vi "Handle Incoming Packets.vi"(8 "error in (no error)":errorcluster, 9 "SessionMailbox":refnum<queue>, 10 "Incoming Packet":refnum<class "ControlPacket.lvclass">, 11 "Client in":refnum<class "Client.lvclass">) -> (0 "error out":errorcluster, 1 "SessionMailbox out":refnum<queue>, 2 "Outgoing":T1, 3 "Client out":refnum<class "Client.lvclass">)   [LabVIEW 2013, in "MQTT Client.lvlib" / "Client.lvclass"]
uses:
  Client.lvclass
  <vilib>/LabVIEW Open Source Project/MQTT Control Packets/Control Packets/ControlPacket/ControlPacket.lvclass
  MQTT_Base/Base Class/Response -- cluster.ctl
  Client.lvclass/Client.ctl
  <vilib>/LabVIEW Open Source Project/MQTT Control Packets/Control Packets/CONNACK/CONNACK.lvclass
  <vilib>/LabVIEW Open Source Project/MQTT Control Packets/Control Packets/CONNACK/Connect Return Code -- enum.ctl
  MQTT_Base/Base Class/MQTT_Base.lvclass
  <vilib>/LabVIEW Open Source Project/MQTT Control Packets/Control Packets/PUBREC/PUBREC.lvclass
  <vilib>/LabVIEW Open Source Project/MQTT Control Packets/Control Packets/PUBLISH/PUBLISH.lvclass
  <vilib>/LabVIEW Open Source Project/MQTT Control Packets/Control Packets/PUBCOMP/PUBCOMP.lvclass
  <vilib>/LabVIEW Open Source Project/MQTT Control Packets/Control Packets/ControlPacket/ControlPacket.lvclass/ControlPacket.ctl
  <vilib>/LabVIEW Open Source Project/MQTT Control Packets/Control Packets/SUBACK/SUBACK.lvclass
  <vilib>/LabVIEW Open Source Project/MQTT Control Packets/Control Packets/UNSUBACK/UNSUBACK.lvclass
  <vilib>/LabVIEW Open Source Project/MQTT Control Packets/Control Packets/PINGRESP/PINGRESP.lvclass
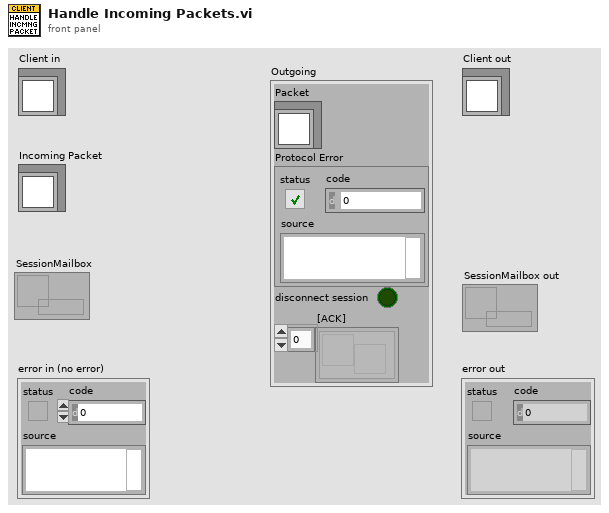
[diagram p1: front panel]
types:
  T1 = typedef "MQTT Base.lvlib/MQTT_Base.lvclass/Response -- cluster.ctl" = cluster{"Packet":refnum<class "ControlPacket.lvclass">, "Protocol Error":errorcluster, "disconnect session":bool, "[ACK]":refnum<notifier>[]}
  T2 = typedef "MQTT_Control_Packets.lvlib/CONNACK.lvclass/Connect Return Code -- enum.ctl" = enum16{"Connection accepted", "Unacceptable protocol version", "Identifier Rejected", "Server Unavailable", "Bad Username or Password", "Not Authorized"}
  T3 = typedef "MQTT_Control_Packets.lvlib/ControlPacket.lvclass/Control Packet Type -- enum.ctl" = enum16{"Reserved", "CONNECT", "CONNACK", "PUBLISH", "PUBACK", "PUBREC", "PUBREL", "PUBCOMP", "SUBSCRIBE", "SUBACK", "UNSUBSCRIBE", "UNSUBACK", "PINGREQ", "PINGRESP", "DISCONNECT", "AUTH"}
  T4 = typedef "MQTT Client.lvlib/Client.lvclass/Public Events -- cluster.ctl" = cluster{"Connection Status":refnum<user-event>, "Connected":refnum<user-event>, "Application Message":refnum<user-event>}
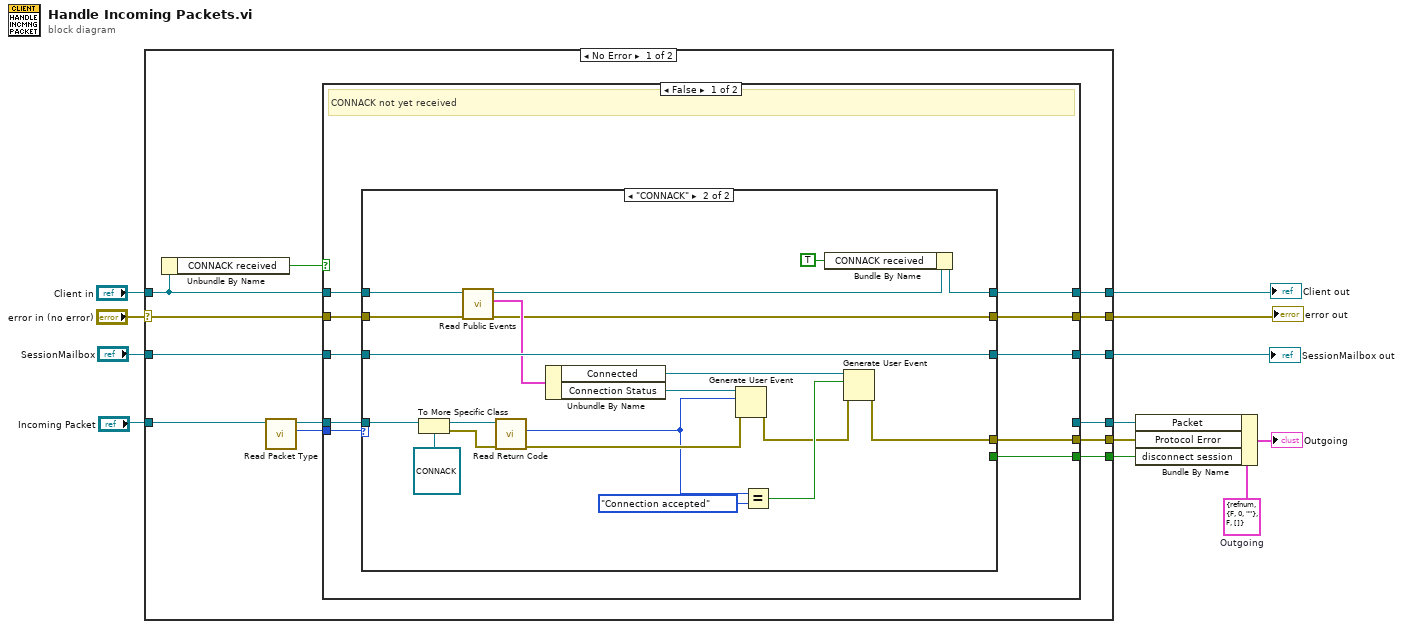
[diagram p0: block diagram]
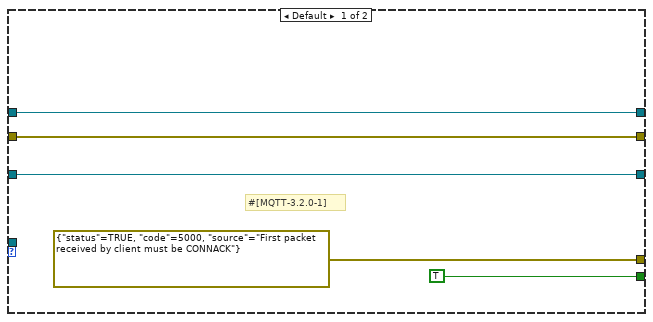
[diagram p2: hidden frame]
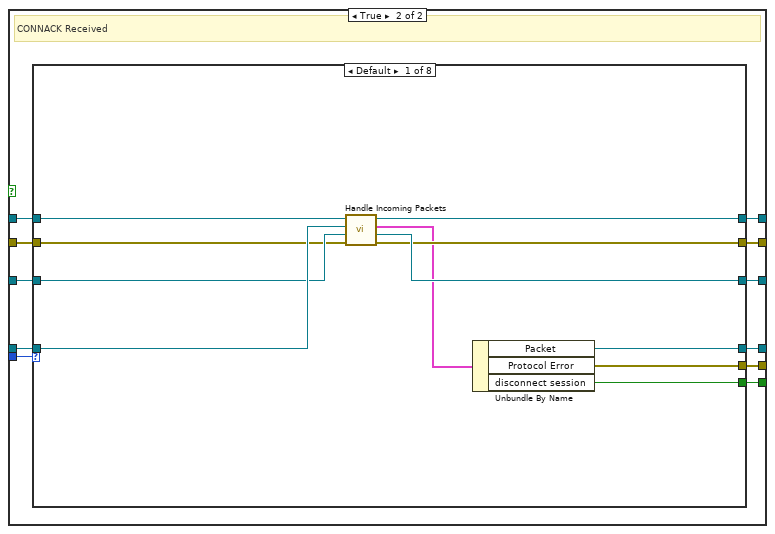
[diagram p3: hidden frame]
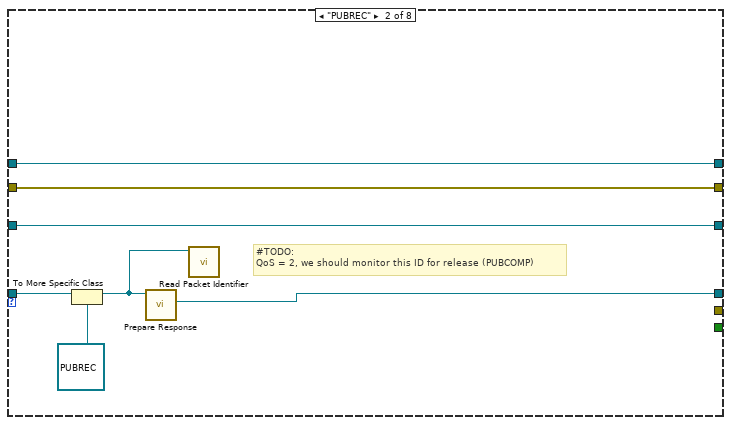
[diagram p4: hidden frame]
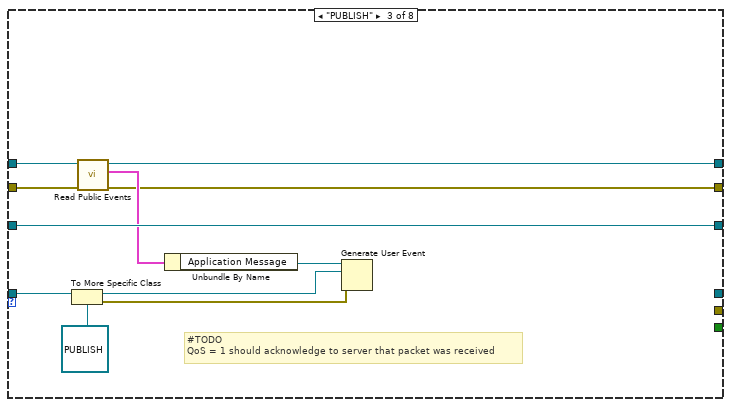
[diagram p5: hidden frame]
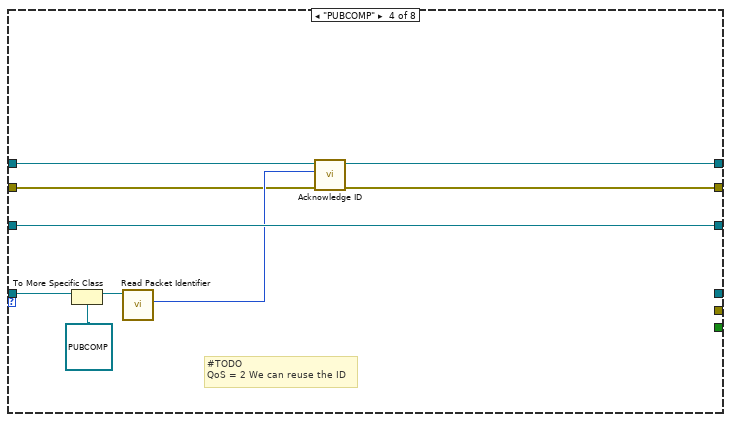
[diagram p6: hidden frame]
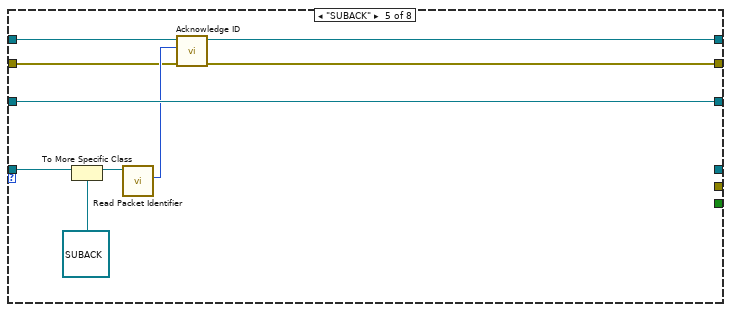
[diagram p7: hidden frame]
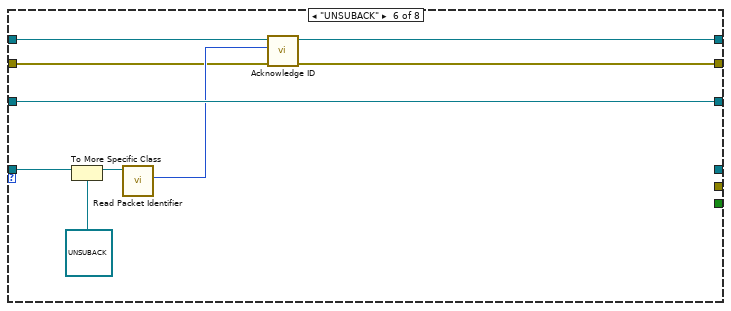
[diagram p8: hidden frame]
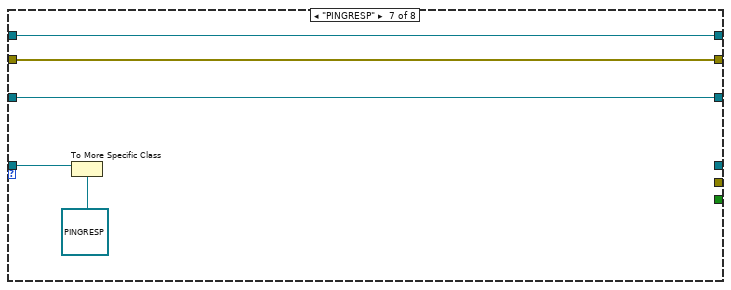
[diagram p9: hidden frame]
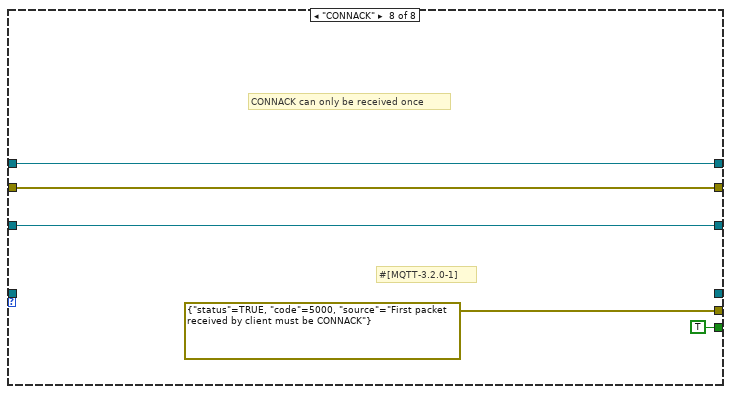
[diagram p10: hidden frame]
diagram:
  w12 = T1 {"Packet"=refnum, "Protocol Error"={"status"=FALSE, "code"=0, "source"=""}, "disconnect session"=FALSE, "[ACK]"=[]}  # Outgoing
  n1 = case shown="No Error" "error in (no error)" {
    selector: "error in (no error)" -> [w23 w140]
    tunnel: [w21 w140] -> w4
    tunnel: [w22 w139] -> w8
    tunnel: "Client in" -> [w14 w139]
    tunnel: "Incoming Packet" -> [w17 _]
    tunnel: [w20 _] -> w1
    tunnel: [w19 _] -> w10
    tunnel: "SessionMailbox" -> [w18 w138]
    tunnel: [w16 w138] -> w3
    tunnel: [w15 _] -> w11
    frame No Error {
      n2 = Unbundle By Name(w14) -> ("CONNACK received"=w13:bool)
      n3 = call <vilib>:"Read Packet Type.vi"("ControlPacket in"=w17) -> ("Control Packet Type"=w25:T3, "ControlPacket out"=w24:refnum<class "ControlPacket.lvclass">)  [unwired: 9 in]
      n4 = case shown="False" w13 {
        tunnel: w25 -> [w32 w71]
        tunnel: w24 -> [w35 w70]
        tunnel: w23 -> [w29 w69]
        tunnel: [w31 w68] -> w22
        tunnel: [w30 w67] -> w21
        tunnel: [_ w66] -> w20
        tunnel: [w34 w65] -> w19
        tunnel: w18 -> [w27 w64]
        tunnel: [w28 w63] -> w16
        tunnel: [w26 w62] -> w15
        tunnel: w14 -> [w33 w61]
        frame False {
          # "CONNACK not yet received"
          n5 = case shown="\"CONNACK\"" w32 {
            tunnel: w35 -> [_ w52]
            tunnel: [errorcluster {"status"=TRUE, "code"=5000, "source"="First packet received by client must be CONNACK"} ("error out 2") w51] -> w34
            tunnel: w33 -> [w40 w44]
            tunnel: [w40 w50] -> w31
            tunnel: [w39 w41] -> w30
            tunnel: w29 -> [w39 w42]
            tunnel: w27 -> [w38 w48]
            tunnel: [w38 w48] -> w28
            tunnel: [TRUE ("status") _] -> w26
            frame Default {
              # "#[MQTT-3.2.0-1]"
            }
            frame "CONNACK" {
              n6 = To More Specific Class(target class=refnum<class "CONNACK.lvclass"> refnum ("CONNACK in"), reference=w52) -> (specific class reference=w59:refnum<class "CONNACK.lvclass">, error out=w58:errorcluster)  [unwired: 1 in]
              n7 = call "Read Public Events.vi"("error in (no error)"=w42, "Client in"=w44) -> ("error out"=w41:errorcluster, "Client Public Events"=w47:T4, "Client out"=w43:refnum<class "Client.lvclass">)  [unwired: 7 in]
              n8 = call <vilib>:"Read Return Code.vi"("error in (no error)"=w58, "CONNACK in"=w59) -> ("error out"=w57:errorcluster, "Return Code"=w56:T2)  [unwired: 7 in, 1 out]
              n9 = Unbundle By Name(w47) -> ("Connected"=w46:refnum<user-event>, "Connection Status"=w45:refnum<user-event>)
              n10 = Generate User Event(user event=w45, event data cluster=w56, error in=w57) -> (error out=w53:errorcluster)  [unwired: 1 in, 1 out]
              n11 = Equal?(x=w56, y=Connect_Return_Code_--_enum."Connection accepted") -> (x = y?=w54:bool)
              n12 = Bundle By Name(cluster=w43, "CONNACK received"=TRUE) -> (w50:refnum<class "Client.lvclass">)
              n13 = Generate User Event(user event=w46, event data cluster=w54, error in=w53) -> (error out=w51:errorcluster)  [unwired: 1 in, 1 out]
            }
          }
        }
        frame True {
          # "CONNACK Received"
          n14 = case shown="Default" w71 {
            tunnel: w70 -> [w82 w86 w99 w108 w117 w126 w129 _]
            tunnel: w69 -> [w77 w88 w93 w102 w113 w120 w131 w137]
            tunnel: w61 -> [w79 w89 w91 w105 w111 w122 w132 w135]
            tunnel: [w78 w89 w90 w104 w110 w121 w132 w135] -> w68
            tunnel: [w76 w88 w92 w101 w112 w119 w131 w137] -> w67
            tunnel: w64 -> [w81 w87 w100 w109 w118 w127 w130 w136]
            tunnel: [w74 w84 _ _ _ _ _ _] -> w66
            tunnel: [w73 _ _ _ _ _ _ errorcluster {"status"=TRUE, "code"=5000, "source"="First packet received by client must be CONNACK"} ("error out 2")] -> w65
            tunnel: [w80 w87 w100 w109 w118 w127 w130 w136] -> w63
            tunnel: [w72 _ _ _ _ _ _ TRUE ("disconnect")] -> w62
            frame Default {
              n15 = call-parent "Handle Incoming Packets.vi"("error in (no error)"=w77, "SessionMailbox"=w81, "Incoming Packet"=w82, "MQTT_Base in"=w79) -> ("error out"=w76:errorcluster, "SessionMailbox out"=w80:refnum<queue>, "Outgoing"=w75:T1, "MQTT_Base out"=w78:refnum<class "Client.lvclass">)  [unwired: 4 in]
              n16 = Unbundle By Name(w75) -> ("Packet"=w74:refnum<class "ControlPacket.lvclass">, "Protocol Error"=w73:errorcluster, "disconnect session"=w72:bool)
            }
            frame "PUBREC" {
              # "#TODO: \nQoS = 2, we should monitor this ID for release (PUBCOMP)"
              n17 = To More Specific Class(target class=refnum<class "PUBREC.lvclass"> refnum ("PUBREC.lvclass"), reference=w86) -> (specific class reference=w83:refnum<class "PUBREC.lvclass">)  [unwired: 1 in, 1 out]
              n18 = call-dynamic "Prepare Response.vi"("PUBREC in"=w83) -> ("ControlPacket response"=w84:refnum<class "ControlPacket.lvclass">)  [unwired: 7 in, 3 out]
              n19 = call <vilib>:"Read Packet Identifier.vi"("ControlPacket in"=w83) -> ()  [unwired: 9 in, 2 out]
            }
            frame "PUBLISH" {
              # "#TODO \nQoS = 1 should acknowledge to server that packet was received"
              n20 = To More Specific Class(target class=refnum<class "PUBLISH.lvclass"> refnum ("PUBLISH.lvclass"), reference=w99) -> (specific class reference=w95:refnum<class "PUBLISH.lvclass">, error out=w94:errorcluster)  [unwired: 1 in]
              n21 = call "Read Public Events.vi"("error in (no error)"=w93, "Client in"=w91) -> ("error out"=w92:errorcluster, "Client Public Events"=w97:T4, "Client out"=w90:refnum<class "Client.lvclass">)  [unwired: 7 in]
              n22 = Unbundle By Name(w97) -> ("Application Message"=w96:refnum<user-event>)
              n23 = Generate User Event(user event=w96, event data cluster=w95, error in=w94) -> ()  [unwired: 1 in, 2 out]
            }
            frame "PUBCOMP" {
              # "#TODO \nQoS = 2 We can reuse the ID"
              n24 = To More Specific Class(target class=refnum<class "PUBCOMP.lvclass"> refnum ("PUBCOMP.lvclass"), reference=w108) -> (specific class reference=w107:refnum<class "PUBCOMP.lvclass">)  [unwired: 1 in, 1 out]
              n25 = call <vilib>:"Read Packet Identifier.vi"("ControlPacket in"=w107) -> ("Packet Identifier"=w103:u16)  [unwired: 9 in, 1 out]
              n26 = call "Acknowledge ID.vi"("error in (no error)"=w102, "Packet Identifier"=w103, "Client in"=w105) -> ("error out"=w101:errorcluster, "Client out"=w104:refnum<class "Client.lvclass">)  [unwired: 7 in]
            }
            frame "SUBACK" {
              n27 = To More Specific Class(target class=refnum<class "SUBACK.lvclass"> refnum ("SUBACK.lvclass"), reference=w117) -> (specific class reference=w116:refnum<class "SUBACK.lvclass">)  [unwired: 1 in, 1 out]
              n28 = call <vilib>:"Read Packet Identifier.vi"("ControlPacket in"=w116) -> ("Packet Identifier"=w114:u16)  [unwired: 9 in, 1 out]
              n29 = call "Acknowledge ID.vi"("error in (no error)"=w113, "Packet Identifier"=w114, "Client in"=w111) -> ("error out"=w112:errorcluster, "Client out"=w110:refnum<class "Client.lvclass">)  [unwired: 7 in]
            }
            frame "UNSUBACK" {
              n30 = To More Specific Class(target class=refnum<class "UNSUBACK.lvclass"> refnum ("UNSUBACK.lvclass"), reference=w126) -> (specific class reference=w125:refnum<class "UNSUBACK.lvclass">)  [unwired: 1 in, 1 out]
              n31 = call <vilib>:"Read Packet Identifier.vi"("ControlPacket in"=w125) -> ("Packet Identifier"=w123:u16)  [unwired: 9 in, 1 out]
              n32 = call "Acknowledge ID.vi"("error in (no error)"=w120, "Packet Identifier"=w123, "Client in"=w122) -> ("error out"=w119:errorcluster, "Client out"=w121:refnum<class "Client.lvclass">)  [unwired: 7 in]
            }
            frame "PINGRESP" {
              n33 = To More Specific Class(target class=refnum<class "PINGRESP.lvclass"> refnum ("PINGRESP.lvclass"), reference=w129) -> ()  [unwired: 1 in, 2 out]
            }
            frame "CONNACK" {
              # "#[MQTT-3.2.0-1]"
              # "CONNACK can only be received once"
            }
          }
        }
      }
    }
    frame Error {
    }
  }
  "error out" <- w4
  "Client out" <- w8
  "SessionMailbox out" <- w3
  n34 = Bundle By Name(cluster=w12, "Packet"=w1, "Protocol Error"=w10, "disconnect session"=w11) -> (→"Outgoing":T1)
